vi "利用组合公式求组合（采用对数扩大取值范围）.vi"(11 "n":i32=100) -> (3 "C(n,k)":dbl)   [LabVIEW 2011]
doc: "功能：\n\n利用组合公式求组合。\n\n公式：\n\nC(n,k)=n!/(k!*(n-k)!\n\n该VI存在下列两个重要的问题，将在其它组合VI中改进：\n1、当阶乘给定超过170时导致阶乘为无穷大，因此限制了计算范围。\n2、直接使用公式导致了大量的重复计算，效率极低。\n\nCSXCS_366创建"
uses:
  <vilib>/gmath/NI_Gmath.lvlib
panel:
  in  "k":i32=100
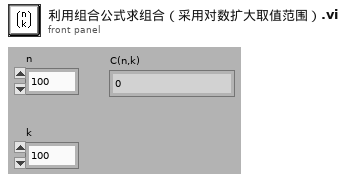
[diagram p1: front panel]
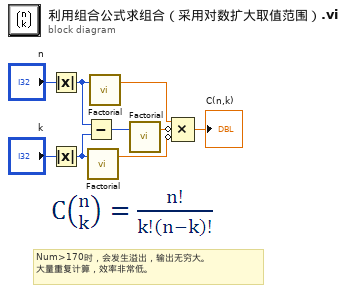
[diagram p0: block diagram]
diagram:
  # "Num>170时，会发生溢出，输出无穷大。\n大量重复计算，效率非常低。"
  n1 = Absolute Value(x="n") -> (abs(x)=w7:i32)
  n2 = Absolute Value(x="k") -> (abs(x)=w6:i32)
  n3 = Subtract(x=w7, y=w6) -> (x-y=w5:i32)
  n4 = call <vilib>:"Factorial.vi"("n"=w6) -> ("n!"=w1:dbl)  [unwired: 2 in]
  n5 = call <vilib>:"Factorial.vi"("n"=w7) -> ("n!"=w4:dbl)  [unwired: 2 in]
  n6 = call <vilib>:"Factorial.vi"("n"=w5) -> ("n!"=w2:dbl)  [unwired: 2 in]
  n7 = Compound Arithmetic op=MULTIPLY(w4, invert w2, invert w1) -> (→"C(n,k)":dbl)
